vi "rsscope_core_global.vi"() -> ()   [LabVIEW 2014] (continued)
you see the signal that would be at the measurement point if the probe&apos;s input impedance is ideal (infinite impedance). Without removing the loading, you see the real signal at the measurement point, including the probe loading.\n\nAvailable Repeated Capabilities:\nChannel: CH1, CH2, CH3, CH4, CHExt\r\n\nRemote-control command(s):\nDEEMbedding<m>:COMPonent<n>:LOAD:REMProbeload"}, {"Level"=2, "Class Only"=FALSE, "Identifier"="RSSCOPE_ATTR_DEEMBEDDING_COMPONENT_IMPEDANCE_TYPE", "Descriptive Name"="Deembedding Component Impedance Type", "Data Type"=0, "Command"="DEEM{Channel}:COMP<Component>:LOAD", "Access"=2, "Range Table"="RsScope_rngDeembeddingComponentImpedanceType", "Read Callback"="rsscope_FormatDeembeddingComponentRepCapInt32_ReadCallback.vi", "Write Callback"="rsscope_FormatDeembeddingComponentRepCapInt32_WriteCallback.vi", "Supported Models"="", "Instrument Options"="K121", "Flags"=0, "Help"="Sets the impedance type of the DUT.\n\nAvailable Repeated Capabilities:\nChannel: CH1, CH2, CH3, CH4, CHExt\r\n\nRemote-control command(s):\nDEEMbedding<m>:COMPonent<n>:LOAD[:TYPE]"}, {"Level"=2, "Class Only"=FALSE, "Identifier"="RSSCOPE_ATTR_DEEMBEDDING_COMPONENT_IMPEDANCE", "Descriptive Name"="Deembedding Component Impedance", "Data Type"=1, "Command"="DEEM{Channel}:COMP<Component>:LOAD:IMP", "Access"=2, "Range Table"="", "Read Callback"="rsscope_FormatDeembeddingComponentRepCapReal64_ReadCallback.vi", "Write Callback"="rsscope_FormatDeembeddingComponentRepCapReal64_WriteCallback.vi", "Supported Models"="", "Instrument Options"="K121", "Flags"=0, "Help"="Impedance of the DUT. Shows the default source impedance or sets the user-defined constant impedance value. If an R&S RT-ZM probe is connected, the value depends on the selected probe mode: common mode, differential, or single-ended measurement.\n\nAvailable Repeated Capabilities:\nChannel: CH1, CH2, CH3, CH4, CHExt\r\n\nRemote-control command(s):\nDEEMbedding<m>:COMPonent<n>:LOAD:IMPedance"}, {"Level"=2, "Class Only"=FALSE, "Identifier"="RSSCOPE_ATTR_DEEMBEDDING_COMPONENT_IDENTICAL_PATHS", "Descriptive Name"="Deembedding Component Identical Paths", "Data Type"=3, "Command"="DEEM{Channel}:COMP<Component>:IDEN", "Access"=2, "Range Table"="", "Read Callback"="rsscope_FormatDeembeddingComponentRepCapBoolean_ReadCallback.vi", "Write Callback"="rsscope_FormatDeembeddingComponentRepCapBoolean_WriteCallback.vi", "Supported Models"="", "Instrument Options"="K121", "Flags"=0, "Help"="The setting is relevant if the measurement setup is a 4-port, and the component is a 2- port. Usually, these components are cables and adapters, which are described by *.s2p files. In case of a 4-port setup, 2 cables or 2 adapters are used. If they are identical, for example, when a matched-pair cable is used, they can be described by the same file. In this case, set the attribute to ON.\n\nAvailable Repeated Capabilities:\nChannel: CH1, CH2, CH3, CH4, CHExt\r\n\nRemote-control command(s):\nDEEMbedding<m>:COMPonent<n>:IDENtical"}, {"Level"=2, "Class Only"=FALSE, "Identifier"="RSSCOPE_ATTR_DEEMBEDDING_COMPONENT_INPUT_PORT_1", "Descriptive Name"="Deembedding Component Input Port 1", "Data Type"=0, "Command"="DEEM{Channel}:COMP<Component>:IPON", "Access"=2, "Range Table"="RsScope_rngDeembeddingComponentPort", "Read Callback"="rsscope_FormatDeembeddingComponentRepCapInt32_ReadCallback.vi", "Write Callback"="rsscope_FormatDeembeddingComponentRepCapInt32_WriteCallback.vi", "Supported Models"="", "Instrument Options"="K121", "Flags"=0, "Help"="Assign the ports to the input 1 of the component according to the data in the Touchstone file. This information is not directly written in the file. You need background information how the S-parameters were determined, i.e. which port was input and which port was output.\n\nAvailable Repeated Capabilities:\nChannel: CH1, CH2, CH3, CH4, CHExt\r\n\nRemote-control command(s):\nDEEMbedding<m>:COMPonent<n>:IPONe"}, {"Level"=2, "Class Only"=FALSE, "Identifier"="RSSCOPE_ATTR_DEEMBEDDING_COMPONENT_INPUT_PORT_2", "Descriptive Name"="Deembedding Component Input Port 2", "Data Type"=0, "Command"="DEEM{Channel}:COMP<Component>:IPTW", "Access"=2, "Range Table"="RsScope_rngDeembeddingComponentPort", "Read Callback"="rsscope_FormatDeembeddingComponentRepCapInt32_ReadCallback.vi", "Write Callback"="rsscope_FormatDeembeddingComponentRepCapInt32_WriteCallback.vi", "Supported Models"="", "Instrument Options"="K121", "Flags"=0, "Help"="Assign the ports to the input 2 of the component according to the data in the Touchstone file. This information is not directly written in the file. You need background information how the S-parameters were determined, i.e. which port was input and which port was output.\n\nAvailable Repeated Capabilities:\nChannel: CH1, CH2, CH3, CH4, CHExt\r\n\nRemote-control command(s):\nDEEMbedding<m>:COMPonent<n>:IPTWo"}, {"Level"=2, "Class Only"=FALSE, "Identifier"="RSSCOPE_ATTR_DEEMBEDDING_COMPONENT_OUTPUT_PORT_1", "Descriptive Name"="Deembedding Component Output Port 1", "Data Type"=0, "Command"="DEEM{Channel}:COMP<Component>:OPON", "Access"=2, "Range Table"="RsScope_rngDeembeddingComponentPort", "Read Callback"="rsscope_FormatDeembeddingComponentRepCapInt32_ReadCallback.vi", "Write Callback"="rsscope_FormatDeembeddingComponentRepCapInt32_WriteCallback.vi", "Supported Models"="", "Instrument Options"="K121", "Flags"=0, "Help"="Assign the ports to the output 1 of the component according to the data in the Touchstone file. This information is not directly written in the file. You need background information how the S-parameters were determined, i.e. which port was input and which port was output.\n\nAvailable Repeated Capabilities:\nChannel: CH1, CH2, CH3, CH4, CHExt\r\n\nRemote-control command(s):\nDEEMbedding<m>:COMPonent<n>:OPONe"}, {"Level"=2, "Class Only"=FALSE, "Identifier"="RSSCOPE_ATTR_DEEMBEDDING_COMPONENT_OUTPUT_PORT_2", "Descriptive Name"="Deembedding Component Output Port 2", "Data Type"=0, "Command"="DEEM{Channel}:COMP<Component>:OPTW", "Access"=2, "Range Table"="RsScope_rngDeembeddingComponentPort", "Read Callback"="rsscope_FormatDeembeddingComponentRepCapInt32_ReadCallback.vi", "Write Callback"="rsscope_FormatDeembeddingComponentRepCapInt32_WriteCallback.vi", "Supported Models"="", "Instrument Options"="K121", "Flags"=0, "Help"="Assign the ports to the output 2 of the component according to the data in the Touchstone file. This information is not directly written in the file. You need background information how the S-parameters were determined, i.e. which port was input and which port was output.\n\nAvailable Repeated Capabilities:\nChannel: CH1, CH2, CH3, CH4, CHExt\r\n\nRemote-control command(s):\nDEEMbedding<m>:COMPonent<n>:OPTWo"}, {"Level"=2, "Class Only"=FALSE, "Identifier"="RSSCOPE_ATTR_DEEMBEDDING_ATTENUATION_DC", "Descriptive Name"="Deembedding Attenuation DC", "Data Type"=1, "Command"="DEEM{Channel}:CADC?", "Access"=0, "Range Table"="", "Read Callback"="", "Write Callback"="", "Supported Models"="", "Instrument Options"="K121", "Flags"=0, "Help"="Maximum attenuation or gain of the measurement setup before deembedding at DC. This value is the expected basic attenuation or gain, which is corrected by deembedding.\n\nAvailable Repeated Capabilities:\nChannel: CH1, CH2, CH3, CH4, CHExt\r\n\nRemote-control command(s):\nDEEMbedding<m>:CADC?"}, {"Level"=2, "Class Only"=FALSE, "Identifier"="RSSCOPE_ATTR_DEEMBEDDING_ATTENUATION_MAX", "Descriptive Name"="Deembedding Attenuation Max", "Data Type"=1, "Command"="DEEM{Channel}:MATT?", "Access"=0, "Range Table"="", "Read Callback"="", "Write Callback"="", "Supported Models"="", "Instrument Options"="K121", "Flags"=0, "Help"="Maximum attenuation of the measurement setup before deembedding, with reference to a frequency response normalized at DC to 0 dB. The deembedding filter must amplify the amplitude response by the &apos;Attmax&apos; value, and thus also increases the noise by this value. The value also helps to decide whether deembedding is useful for the defined effective bandwidth.\n\nAvailable Repeated Capabilities:\nChannel: CH1, CH2, CH3, CH4, CHExt\r\n\nRemote-control command(s):\nDEEMbedding<m>:MATTenuation?"}, {"Level"=2, "Class Only"=FALSE, "Identifier"="RSSCOPE_ATTR_DEEMBEDDING_GAIN_MAX", "Descriptive Name"="Deembedding Gain Max", "Data Type"=1, "Command"="DEEM{Channel}:MGA?", "Access"=0, "Range Table"="", "Read Callback"="", "Write Callback"="", "Supported Models"="", "Instrument Options"="K121", "Flags"=0, "Help"="Maximum gain of the measurement setup before deembedding, with reference to a frequency response normalized at DC to 0dB. The deembedding filter must attenuate the amplitude response by this value. The value helps also to avoid an overload of the ADC.\n\nAvailable Repeated Capabilities:\nChannel: CH1, CH2, CH3, CH4, CHExt\r\n\nRemote-control command(s):\nDEEMbedding<m>:MGAin?"}, {"Level"=1, "Class Only"=TRUE, "Identifier"="", "Descriptive Name"="Mixed Signal Option (MSO)", "Data Type"=0, "Command"="", "Access"=0, "Range Table"="", "Read Callback"="", "Write Callback"="", "Supported Models"="", "Instrument Options"="", "Flags"=0, "Help"="The Mixed Signal Option R&S RTO-B1 adds logic analyzer functions to the classical\noscilloscope functions. Using the MSO option, you can analyze and debug embedded\nsystems with mixed-signal designs that use analog signals and correlated digital signals\nsimultaneously."}, {"Level"=2, "Class Only"=TRUE, "Identifier"="", "Descriptive Name"="Trigger", "Data Type"=0, "Command"="", "Access"=0, "Range Table"="", "Read Callback"="", "Write Callback"="", "Supported Models"="", "Instrument Options"="", "Flags"=0, "Help"="MSO trigger settings."}, {"Level"=3, "Class Only"=FALSE, "Identifier"="RSSCOPE_ATTR_MSO_TRIGGER_TYPE", "Descriptive Name"="MSO Trigger Type", "Data Type"=0, "Command"="TRIG:PAR:TYPE", "Access"=2, "Range Table"="rsscope_rngMSOTriggerType", "Read Callback"="", "Write Callback"="", "Supported Models"="", "Instrument Options"="B1", "Flags"=0, "Help"="Sets the MSO trigger type.\n\nAvailable Repeated Capabilities:\nNone\n\nRemote-control command(s):\nTRIGger<m>:PARallel:TYPE"}, {"Level"=3, "Class Only"=FALSE, "Identifier"="RSSCOPE_ATTR_MSO_TRIGGER_SOURCE", "Descriptive Name"="MSO Trigger Source", "Data Type"=0, "Command"="TRIG:SOUR", "Access"=2, "Range Table"="rsscope_rngMSOTriggerSource", "Read Callback"="", "Write Callback"="", "Supported Models"="", "Instrument Options"="B1", "Flags"=0, "Help"="Sets the trigger source for the selected trigger type.\n\nAvailable Repeated Capabilities:\nNone\n\nRemote-control command(s):\nTRIGger<m>:SOURce[:SELect]"}, {"Level"=3, "Class Only"=TRUE, "Identifier"="", "Descriptive Name"="Edge", "Data Type"=0, "Command"="", "Access"=0, "Range Table"="", "Read Callback"="", "Write Callback"="", "Supported Models"="", "Instrument Options"="", "Flags"=0, "Help"="MSO trigger edge settings."}, {"Level"=4, "Class Only"=FALSE, "Identifier"="RSSCOPE_ATTR_MSO_EDGE_TRIGGER_EXPRESSION", "Descriptive Name"="MSO Edge Trigger Expression", "Data Type"=2, "Command"="TRIGger1:PAR:EDGE:EXPR", "Access"=2, "Range Table"="", "Read Callback"="", "Write Callback"="", "Supported Models"="", "Instrument Options"="B1", "Flags"=0, "Help"="Defines a logical combination of several digital channels as trigger condition.\n\nExample: &apos;D1 and D2&apos;\n\nAvailable Repeated Capabilities:\nNone\n\nRemote-control command(s):\nTRIGger<m>:PARallel:EDGE:EXPRession[:DEFine]"}, {"Level"=4, "Class Only"=FALSE, "Identifier"="RSSCOPE_ATTR_MSO_EDGE_TRIGGER_SLOPE", "Descriptive Name"="MSO Edge Trigger Slope", "Data Type"=0, "Command"="TRIG:PAR:EDGE:SLOP", "Access"=2, "Range Table"="rsscope_rngTriggerSlope", "Read Callback"="", "Write Callback"="", "Supported Models"="", "Instrument Options"="B1", "Flags"=0, "Help"="Defines the edge - the state transition - of the signal to trigger on a single digital channel (a logic bit), or a logical combination of digital channels.\n\nAvailable Repeated Capabilities:\nNone\n\nRemote-control command(s):\nTRIGger<m>:PARallel:EDGE:SLOPe"}, {"Level"=3, "Class Only"=TRUE, "Identifier"="", "Descriptive Name"="Width", "Data Type"=0, "Command"="", "Access"=0, "Range Table"="", "Read Callback"="", "Write Callback"="", "Supported Models"="", "Instrument Options"="", "Flags"=0, "Help"="MSO trigger width settings."}, {"Level"=4, "Class Only"=FALSE, "Identifier"="RSSCOPE_ATTR_MSO_WIDTH_TRIGGER_EXPRESSION", "Descriptive Name"="MSO Width Trigger Expression", "Data Type"=2, "Command"="TRIGger1:PAR:WIDT:EXPR", "Access"=2, "Range Table"="", "Read Callback"="", "Write Callback"="", "Supported Models"="", "Instrument Options"="B1", "Flags"=0, "Help"="Defines a logical combination of several digital channels as trigger condition.\n\nExample: &apos;D1 and D2&apos;\n\nAvailable Repeated Capabilities:\nNone\n\nRemote-control command(s):\nTRIGger<m>:PARallel:WIDTh:EXPRession[:DEFine]"}, {"Level"=4, "Class Only"=FALSE, "Identifier"="RSSCOPE_ATTR_MSO_WIDTH_TRIGGER_POLARITY", "Descriptive Name"="MSO Width Trigger Polarity", "Data Type"=0, "Command"="TRIGger1:PAR:WIDT:POL", "Access"=2, "Range Table"="rsscope_rngTriggerSlope", "Read Callback"="", "Write Callback"="", "Supported Models"="", "Instrument Options"="B1", "Flags"=0, "Help"="Sets the polarity of the pulse. When triggering on a positive pulse, the trigger event occurs on the high to low transition of the pulse if the timing condition is true. When triggering on a negative pulse, the trigger event occurs on the low to high transition of the pulse if the timing condition is true.\n\nAvailable Repeated Capabilities:\nNone\n\nRemote-control command(s):\nTRIGger<m>:PARallel:WIDTh:POLarity"}, {"Level"=4, "Class Only"=FALSE, "Identifier"="RSSCOPE_ATTR_MSO_WIDTH_TRIGGER_CONDITION", "Descriptive Name"="MSO Width Trigger Condition", "Data Type"=0, "Command"="TRIGger1:PAR:WIDT:RANG", "Access"=2, "Range Table"="rsscope_rngWidthCondition", "Read Callback"="", "Write Callback"="", "Supported Models"="", "Instrument Options"="B1", "Flags"=0, "Help"="Selects how the range of a pulse width is defined.\n\nAvailable Repeated Capabilities:\nNone\n\nRemote-control command(s):\nTRIGger<m>:PARallel:WIDTh:RANGe"}, {"Level"=4, "Class Only"=FALSE, "Identifier"="RSSCOPE_ATTR_MSO_WIDTH_TRIGGER_WIDTH", "Descriptive Name"="MSO Width Trigger Width", "Data Type"=1, "Command"="TRIGger1:PAR:WIDT:WIDT", "Access"=2, "Range Table"="rsscope_rngMSOWidth", "Read Callback"="", "Write Callback"="", "Supported Models"="", "Instrument Options"="B1", "Flags"=0, "Help"="For the ranges &apos;Within&apos; and &apos;Outside&apos;, the width defines the center of a range which is defined by the limits &apos;+/-Delta&apos;. For the ranges &apos;Shorter&apos; and &apos;Longer&apos;, the width defines the maximum and minimum pulse width, respectively.\n\nAvailable Repeated Capabilities:\nNone\n\nRemote-control command(s):\nTRIGger<m>:PARallel:WIDTh:WIDTh"}, {"Level"=4, "Class Only"=FALSE, "Identifier"="RSSCOPE_ATTR_MSO_WIDTH_TRIGGER_DELTA", "Descriptive Name"="MSO Width Trigger Delta", "Data Type"=1, "Command"="TRIGger1:PAR:WIDT:DELT", "Access"=2, "Range Table"="rsscope_rngMSOWidthDelta", "Read Callback"="", "Write Callback"="", "Supported Models"="", "Instrument Options"="B1", "Flags"=0, "Help"="Defines a range around the width value.\n\nAvailable Repeated Capabilities:\nNone\n\nRemote-control command(s):\nTRIGger<m>:PARallel:WIDTh:DELTa"}, {"Level"=3, "Class Only"=TRUE, "Identifier"="", "Descriptive Name"="Timeout", "Data Type"=0, "Command"="", "Access"=0, "Range Table"="", "Read Callback"="", "Write Callback"="", "Supported Models"="", "Instrument Options"="", "Flags"=0, "Help"="MSO trigger timeout settings."}, {"Level"=4, "Class Only"=FALSE, "Identifier"="RSSCOPE_ATTR_MSO_TIMEOUT_TRIGGER_EXPRESSION", "Descriptive Name"="MSO Timeout Trigger Expression", "Data Type"=2, "Command"="TRIGger1:PAR:TIM:EXPR", "Access"=2, "Range Table"="", "Read Callback"="", "Write Callback"="", "Supported Models"="", "Instrument Options"="B1", "Flags"=0, "Help"="Defines a logical combination of several digital channels as trigger condition.\n\nExample: &apos;D1 and D2&apos;\n\nAvailable Repeated Capabilities:\nNone\n\nRemote-control command(s):\nTRIGger<m>:PARallel:TIMeout:EXPRession[:DEFine]"}, {"Level"=4, "Class Only"=FALSE, "Identifier"="RSSCOPE_ATTR_MSO_TIMEOUT_TRIGGER_VALUE", "Descriptive Name"="MSO Timeout Trigger Value", "Data Type"=1, "Command"="TRIGger1:PAR:TIM:TIME", "Access"=2, "Range Table"="rsscope_rngMSOTimeoutPattern", "Read Callback"="", "Write Callback"="", "Supported Models"="", "Instrument Options"="B1", "Flags"=0, "Help"="Defines the time limit for the timeout at which the instrument triggers.\n\nAvailable Repeated Capabilities:\nNone\n\nRemote-control command(s):\nTRIGger<m>:PARallel:TIMeout:TIME"}, {"Level"=4, "Class Only"=FALSE, "Identifier"="RSSCOPE_ATTR_MSO_TIMEOUT_TRIGGER_CONDITION", "Descriptive Name"="MSO Timeout Trigger Condition", "Data Type"=0, "Command"="TRIGger1:PAR:TIM:RANG", "Access"=2, "Range Table"="rsscope_rngMSOTimeoutCondition", "Read Callback"="", "Write Callback"="", "Supported Models"="", "Instrument Options"="B1", "Flags"=0, "Help"="Defines the relation of the signal level to the trigger level.\n\nAvailable Repeated Capabilities:\nNone\n\nRemote-control command(s):\nTRIGger<m>:PARallel:TIMeout:RANGe"}, {"Level"=3, "Class Only"=TRUE, "Identifier"="", "Descriptive Name"="Data2Clock", "Data Type"=0, "Command"="", "Access"=0, "Range Table"="", "Read Callback"="", "Write Callback"="", "Supported Models"="", "Instrument Options"="", "Flags"=0, "Help"="MSO trigger Data2Clock settings."}, {"Level"=4, "Class Only"=FALSE, "Identifier"="RSSCOPE_ATTR_MSO_DATA2CLOCK_TRIGGER_CLOCK_SOURCE", "Descriptive Name"="MSO Data2Clock Trigger Clock Source", "Data Type"=0, "Command"="TRIG1:PAR:SETH:CSO", "Access"=2, "Range Table"="rsscope_rngMSOClockSource", "Read Callback"="", "Write Callback"="", "Supported Models"="", "Instrument Options"="B1", "Flags"=0, "Help"="Sets the clock signal source.\n\nAvailable Repeated Capabilities:\nNone\n\nRemote-control command(s):\nTRIGger<m>:PARallel:SETHold:CSOurce[:VALue]"}, {"Level"=4, "Class Only"=FALSE, "Identifier"="RSSCOPE_ATTR_MSO_DATA2CLOCK_TRIGGER_CLOCK_EDGE", "Descriptive Name"="MSO Data2Clock Trigger Clock Edge", "Data Type"=0, "Command"="TRIG1:PAR:SETH:CSO:EDGE", "Access"=2, "Range Table"="rsscope_rngTriggerSlope", "Read Callback"="", "Write Callback"="", "Supported Models"="", "Instrument Options"="B1", "Flags"=0, "Help"="Sets the edge of the clock signal to define the time reference point for the setup and hold time.\n\nAvailable Repeated Capabilities:\nNone\n\nRemote-control command(s):\nTRIGger<m>:PARallel:SETHold:CSOurce:EDGE"}, {"Level"=4, "Class Only"=FALSE, "Identifier"="RSSCOPE_ATTR_MSO_DATA2CLOCK_TRIGGER_HOLD_TIME", "Descriptive Name"="MSO Data2Clock Trigger Hold Time", "Data Type"=1, "Command"="TRIG1:PAR:SETH:HTIM", "Access"=2, "Range Table"="rsscope_rngMSOData2ClockTime", "Read Callback"="", "Write Callback"="", "Supported Models"="", "Instrument Options"="B1", "Flags"=0, "Help"="Sets the minimum time after the clock edge while the data signal must stay steady above or below the data level. The hold time can be negative. In this case, the setup time is always positive. The setup/hold interval starts before the clock edge (setup time) and ends before the clock edge (hold time). If you change the negative hold time, the setup time is adjusted by the intrument.\n\nAvailable Repeated Capabilities:\nNone\n\nRemote-control command(s):\nTRIGger<m>:PARallel:SETHold:HTIMe"}, {"Level"=4, "Class Only"=FALSE, "Identifier"="RSSCOPE_ATTR_MSO_DATA2CLOCK_TRIGGER_SETUP_TIME", "Descriptive Name"="MSO Data2Clock Trigger SetupTime", "Data Type"=1, "Command"="TRIG1:PAR:SETH:STIM", "Access"=2, "Range Table"="rsscope_rngMSOData2ClockTime", "Read Callback"="", "Write Callback"="", "Supported Models"="", "Instrument Options"="B1", "Flags"=0, "Help"="Sets the minimum time before the clock edge while the data signal must stay steady above or below the data level. The setup time can be negative. In this case, the hold time is always positive. The setup/hold interval starts after the clock edge (setup time) and ends after the clock edge (hold time). If you change the negative setup time, the hold time is adjusted by the intrument.\n\nAvailable Repeated Capabilities:\nNone\n\nRemote-control command(s):\nTRIGger<m>:PARallel:SETHold:STIMe"}, {"Level"=3, "Class Only"=TRUE, "Identifier"="", "Descriptive Name"="State", "Data Type"=0, "Command"="", "Access"=0, "Range Table"="", "Read Callback"="", "Write Callback"="", "Supported Models"="", "Instrument Options"="", "Flags"=0, "Help"="MSO trigger state settings."}, {"Level"=4, "Class Only"=FALSE, "Identifier"="RSSCOPE_ATTR_MSO_STATE_TRIGGER_EXPRESSION", "Descriptive Name"="MSO State Trigger Expression", "Data Type"=2, "Command"="TRIGger1:PAR:STAT:EXPR", "Access"=2, "Range Table"="", "Read Callback"="", "Write Callback"="", "Supported Models"="", "Instrument Options"="B1", "Flags"=0, "Help"="Defines a logical combination of several digital channels as trigger condition.\n\nExample: &apos;D1 and D2&apos;\n\nAvailable Repeated Capabilities:\nNone\n\nRemote-control command(s):\nTRIGger<m>:PARallel:STATe:EXPRession[:DEFine]"}, {"Level"=4, "Class Only"=FALSE, "Identifier"="RSSCOPE_ATTR_MSO_STATE_TRIGGER_CLOCK_SOURCE", "Descriptive Name"="MSO State Trigger Clock Source", "Data Type"=0, "Command"="TRIGger1:PAR:STAT:CSO:VAL", "Access"=2, "Range Table"="rsscope_rngMSOClockSource", "Read Callback"="", "Write Callback"="", "Supported Models"="", "Instrument Options"="B1", "Flags"=0, "Help"="Sets the clock signal source.\n\nAvailable Repeated Capabilities:\nNone\n\nRemote-control command(s):\nTRIGger<m>:PARallel:STATe:CSOurce:VALue"}, {"Level"=4, "Class Only"=FALSE, "Identifier"="RSSCOPE_ATTR_MSO_STATE_TRIGGER_CLOCK_EDGE", "Descriptive Name"="MSO State Trigger Clock Edge", "Data Type"=0, "Command"="TRIGger1:PAR:STAT:CSO:EDGE", "Access"=2, "Range Table"="rsscope_rngTriggerSlope", "Read Callback"="", "Write Callback"="", "Supported Models"="", "Instrument Options"="B1", "Flags"=0, "Help"="Sets the edge of the clock signal. The crossing of the clock edge and the logical threshold defines the time at which the logical states and the bus value are analyzed.\n\nAvailable Repeated Capabilities:\nNone\n\nRemote-control command(s):\nTRIGger<m>:PARallel:STATe:CSOurce:EDGE"}, {"Level"=4, "Class Only"=TRUE, "Identifier"="", "Descriptive Name"="Digital Channel", "Data Type"=0, "Command"="", "Access"=0, "Range Table"="", "Read Callback"="", "Write Callback"="", "Supported Models"="", "Instrument Options"="", "Flags"=0, "Help"="MSO trigger state digital channel settings."}, {"Level"=5, "Class Only"=FALSE, "Identifier"="RSSCOPE_ATTR_MSO_STATE_TRIGGER_CHANNEL_STATUS_BIT", "Descriptive Name"="MSO State Trigger Channel Status Bit", "Data Type"=0, "Command"="TRIGger1:PAR:STAT:BIT{DigitalChannel}", "Access"=2, "Range Table"="rsscope_rngMSOTriggerChannelState", "Read Callback"="", "Write Callback"="", "Supported Models"="", "Instrument Options"="B1", "Flags"=0, "Help"="Sets the required state for each digital channel that is used in the bus.\n\nAvailable Repeated Capabilities:\nDigitalChannel: D0, D1, D2, D3, D4, D5, D6, D7, D8, D9, D10, D11, D12, D13, D14, D15\r\n\nRemote-control command(s):\nTRIGger<m>:PARallel:STATe:BIT<n>"}, {"Level"=3, "Class Only"=TRUE, "Identifier"="", "Descriptive Name"="Pattern", "Data Type"=0, "Command"="", "Access"=0, "Range Table"="", "Read Callback"="", "Write Callback"="", "Supported Models"="", "Instrument Options"="", "Flags"=0, "Help"="MSO trigger patern settings."}, {"Level"=4, "Class Only"=FALSE, "Identifier"="RSSCOPE_ATTR_MSO_PATTERN_TRIGGER_EXPRESSION", "Descriptive Name"="MSO Pattern Trigger Expression", "Data Type"=2, "Command"="TRIGger1:PAR:PATT:EXPR", "Access"=2, "Range Table"="", "Read Callback"="", "Write Callback"="", "Supported Models"="", "Instrument Options"="B1", "Flags"=0, "Help"="Defines a logical combination of several digital channels as trigger condition.\n\nExample: &apos;D1 and D2&apos;\n\nAvailable Repeated Capabilities:\nNone\n\nRemote-control command(s):\nTRIGger<m>:PARallel:PATTern:EXPRession[:DEFine]"}, {"Level"=4, "Class Only"=FALSE, "Identifier"="RSSCOPE_ATTR_MSO_PATTERN_TRIGGER_MODE", "Descriptive Name"="MSO Pattern Trigger Mode", "Data Type"=0, "Command"="TRIGger1:PAR:PATT:MODE", "Access"=2, "Range Table"="rsscope_rngMSOPatternMode", "Read Callback"="", "Write Callback"="", "Supported Models"="", "Instrument Options"="B1", "Flags"=0, "Help"="Sets the mode of the timing condition.\n\nAvailable Repeated Capabilities:\nNone\n\nRemote-control command(s):\nTRIGger<m>:PARallel:PATTern:MODE"}, {"Level"=4, "Class Only"=FALSE, "Identifier"="RSSCOPE_ATTR_MSO_PATTERN_TRIGGER_TIMEOUT_MODE", "Descriptive Name"="MSO Pattern Trigger Timeout Mode", "Data Type"=0, "Command"="TRIGger1:PAR:PATT:TIM:MODE", "Access"=2, "Range Table"="rsscope_rngMSOPatternTimeoutMode", "Read Callback"="", "Write Callback"="", "Supported Models"="", "Instrument Options"="B1", "Flags"=0, "Help"="Sets the state condition for the timeout qualification.\n\nAvailable Repeated Capabilities:\nNone\n\nRemote-control command(s):\nTRIGger<m>:PARallel:PATTern:TIMeout:MODE"}, {"Level"=4, "Class Only"=FALSE, "Identifier"="RSSCOPE_ATTR_MSO_PATTERN_TRIGGER_TIMEOUT", "Descriptive Name"="MSO Pattern Trigger Timeout", "Data Type"=1, "Command"="TRIGger1:PAR:PATT:TIM", "Access"=2, "Range Table"="rsscope_rngMSOTimeoutPattern", "Read Callback"="", "Write Callback"="", "Supported Models"="", "Instrument Options"="B1", "Flags"=0, "Help"="Defines how long the result of the pattern condition must be true or false.\n\nAvailable Repeated Capabilities:\nNone\n\nRemote-control command(s):\nTRIGger<m>:PARallel:PATTern:TIMeout[:TIME]"}, {"Level"=4, "Class Only"=FALSE, "Identifier"="RSSCOPE_ATTR_MSO_PATTERN_TRIGGER_WIDTH", "Descriptive Name"="MSO Pattern Trigger Width", "Data Type"=1, "Command"="TRIGger1:PAR:PATT:WIDT", "Access"=2, "Range Table"="rsscope_rngMSOTimeoutPattern", "Read Callback"="", "Write Callback"="", "Supported Models"="", "Instrument Options"="B1", "Flags"=0, "Help"="For the ranges &apos;Within&apos; and &apos;Outside&apos;, the width defines the center of a range which is defined by the limits &apos;Delta&apos;.\nFor the ranges &apos;Shorter&apos; and &apos;Longer&apos;, the width defines the maximum and minimum pulse width, respectively.\n\nAvailable Repeated Capabilities:\nNone\n\nRemote-control command(s):\nTRIGger<m>:PARallel:PATTern:WIDTh[:WIDTh]"}, {"Level"=4, "Class Only"=FALSE, "Identifier"="RSSCOPE_ATTR_MSO_PATTERN_TRIGGER_DELTA", "Descriptive Name"="MSO Pattern Trigger Delta", "Data Type"=1, "Command"="TRIGger1:PAR:PATT:WIDT:DELT", "Access"=2, "Range Table"="rsscope_rngMSOWidthDelta", "Read Callback"="", "Write Callback"="", "Supported Models"="", "Instrument Options"="B1", "Flags"=0, "Help"="Defines how the range of a pulse width is defined for keeping up the true result of the pattern condition.\n\nAvailable Repeated Capabilities:\nNone\n\nRemote-control command(s):\nTRIGger<m>:PARallel:PATTern:WIDTh:DELTa"}, {"Level"=4, "Class Only"=FALSE, "Identifier"="RSSCOPE_ATTR_MSO_PATTERN_TRIGGER_CONDITION", "Descriptive Name"="MSO Pattern Trigger Condition", "Data Type"=0, "Command"="TRIGger1:PAR:PATT:WIDT:RANG", "Access"=2, "Range Table"="rsscope_rngWidthCondition", "Read Callback"="", "Write Callback"="", "Supported Models"="", "Instrument Options"="B1", "Flags"=0, "Help"="Defines how the range of a pulse width is defined for keeping up the true result of the pattern condition.\n\nAvailable Repeated Capabilities:\nNone\n\nRemote-control command(s):\nTRIGger<m>:PARallel:PATTern:WIDTh:RANGe"}, {"Level"=4, "Class Only"=TRUE, "Identifier"="", "Descriptive Name"="Digital Channel", "Data Type"=0, "Command"="", "Access"=0, "Range Table"="", "Read Callback"="", "Write Callback"="", "Supported Models"="", "Instrument Options"="", "Flags"=0, "Help"="MSO trigger patern digital channel settings."}, {"Level"=5, "Class Only"=FALSE, "Identifier"="RSSCOPE_ATTR_MSO_PATTERN_TRIGGER_CHANNEL_STATUS_BIT", "Descriptive Name"="MSO Pattern Trigger Channel Status Bit", "Data Type"=0, "Command"="TRIGger1:PAR:PATT:BIT{DigitalChannel}", "Access"=2, "Range Table"="rsscope_rngMSOTriggerChannelState", "Read Callback"="", "Write Callback"="", "Supported Models"="", "Instrument Options"="B1", "Flags"=0, "Help"="Sets the required state for each digital channel that is used in the bus.\n\nAvailable Repeated Capabilities:\nDigitalChannel: D0, D1, D2, D3, D4, D5, D6, D7, D8, D9, D10, D11, D12, D13, D14, D15\r\n\nRemote-control command(s):\nTRIGger<m>:PARallel:PATTern:BIT<n>"}, {"Level"=3, "Class Only"=TRUE, "Identifier"="", "Descriptive Name"="Serial Pattern", "Data Type"=0, "Command"="", "Access"=0, "Range Table"="", "Read Callback"="", "Write Callback"="", "Supported Models"="", "Instrument Options"="", "Flags"=0, "Help"="MSO trigger serial pattern settings."}, {"Level"=4, "Class Only"=FALSE, "Identifier"="RSSCOPE_ATTR_MSO_SERIAL_PATTERN_TRIGGER_EXPRESSION", "Descriptive Name"="MSO Serial Pattern Trigger Expression", "Data Type"=2, "Command"="TRIGger1:PAR:SPAT:EXPR", "Access"=2, "Range Table"="", "Read Callback"="", "Write Callback"="", "Supported Models"="", "Instrument Options"="B1", "Flags"=0, "Help"="Defines a logical combination of several digital channels as trigger condition.\n\nExample: &apos;D1 and D2&apos;\n\nAvailable Repeated Capabilities:\nNone\n\nRemote-control command(s):\nTRIGger<m>:PARallel:SPATtern:EXPRession[:DEFine]"}, {"Level"=4, "Class Only"=FALSE, "Identifier"="RSSCOPE_ATTR_MSO_SERIAL_PATTERN_TRIGGER_CLOCK_SOURCE", "Descriptive Name"="MSO Serial Pattern Trigger Clock Source", "Data Type"=0, "Command"="TRIGger1:PAR:SPAT:CSO:VAL", "Access"=2, "Range Table"="rsscope_rngMSOClockSource", "Read Callback"="", "Write Callback"="", "Supported Models"="", "Instrument Options"="B1", "Flags"=0, "Help"="Sets the clock signal source.\n\nAvailable Repeated Capabilities:\nNone\n\nRemote-control command(s):\nTRIGger<m>:PARallel:SPATtern:CSOurce[:VALue]"}, {"Level"=4, "Class Only"=FALSE, "Identifier"="RSSCOPE_ATTR_MSO_SERIAL_PATTERN_TRIGGER_CLOCK_EDGE", "Descriptive Name"="MSO Serial Pattern Trigger Clock Edge", "Data Type"=0, "Command"="TRIGger1:PAR:SPAT:CSO:EDGE", "Access"=2, "Range Table"="rsscope_rngTriggerSlope", "Read Callback"="", "Write Callback"="", "Supported Models"="", "Instrument Options"="B1", "Flags"=0, "Help"="The clock edge defines the point in time when the state of the data signal is checked.\n\nAvailable Repeated Capabilities:\nNone\n\nRemote-control command(s):\nTRIGger<m>:PARallel:SPATtern:CSOurce:EDGE"}, {"Level"=4, "Class Only"=FALSE, "Identifier"="RSSCOPE_ATTR_MSO_SERIAL_PATTERN_TRIGGER_PATTERN", "Descriptive Name"="MSO Serial Pattern Trigger Pattern", "Data Type"=2, "Command"="TRIGger1:PAR:SPAT:PATT", "Access"=2, "Range Table"="", "Read Callback"="", "Write Callback"="", "Supported Models"="", "Instrument Options"="", "Flags"=0, "Help"="The pattern contains the bits of the serial data to be found in the data stream. The maximum length of the pattern is 128 bit. You can enter the pattern in binary or hexadecimal format.\n\nAvailable Repeated Capabilities:\nNone\n\nRemote-control command(s):\nTRIGger<m>:PARallel:SPATtern:PATTern"}, {"Level"=2, "Class Only"=TRUE, "Identifier"="", "Descriptive Name"="Digital Channel", "Data Type"=0, "Command"="", "Access"=0, "Range Table"="", "Read Callback"="", "Write Callback"="", "Supported Models"="", "Instrument Options"="", "Flags"=0, "Help"="Selects Digital Channel."}, {"Level"=3, "Class Only"=FALSE, "Identifier"="RSSCOPE_ATTR_MSO_SIGNAL_LABEL", "Descriptive Name"="MSO Signal Label", "Data Type"=2, "Command"="DIG{DigitalChannel}:LAB", "Access"=2, "Range Table"="", "Read Callback"="", "Write Callback"="", "Supported Models"="", "Instrument Options"="B1", "Flags"=0, "Help"="Selects and configure the digital channels that are used in the selected bus.\n\nAvailable Repeated Capabilities:\nDigitalChannel: D0, D1, D2, D3, D4, D5, D6, D7, D8, D9, D10, D11, D12, D13, D14, D15\r\n\nRemote-control command(s):\nDIGital<m>:LABel"}, {"Level"=3, "Class Only"=FALSE, "Identifier"="RSSCOPE_ATTR_MSO_DIGITAL_CHANNEL_DISPLAY", "Descriptive Name"="MSO Digital Channel Display", "Data Type"=3, "Command"="DIG{DigitalChannel}:DISP", "Access"=2, "Range Table"="", "Read Callback"="", "Write Callback"="", "Supported Models"="", "Instrument Options"="", "Flags"=0, "Help"="Enables or disables the indicated digital channel, displays it, and enables the parallel Bus1 if the bus was disabled. That is, RSSCOPE_ATTR_MSO_DISPLAY_SHOW_DIGITAL_SIGNALS and RSSCOPE_ATTR_MSO_BUS_STATE are set to ON automatically.\n\nIf another active bus already uses the selected digital channel, the instrument disables the other bus to avoid conflicts.\nFor Bus1, the DIG:DISP command has the same effect as RSSCOPE_ATTR_MSO_SIGNAL_ASSIGN_STATE. To enable digital channels for buses 2, 3 and 4, use the RSSCOPE_ATTR_MSO_SIGNAL_ASSIGN_STATE command.\n\nAvailable Repeated Capabilities:\nDigitalChannel: D0, D1, D2, D3, D4, D5, D6, D7, D8, D9, D10, D11, D12, D13, D14, D15\r\n\nRemote-control command(s):\nDIGital<m>:DISPlay"}, {"Level"=3, "Class Only"=FALSE, "Identifier"="RSSCOPE_ATTR_MSO_SIGNAL_DESKEW", "Descriptive Name"="MSO Signal Deskew", "Data Type"=1, "Command"="DIG{DigitalChannel}:DESK", "Access"=2, "Range Table"="rsscope_rngMSOSignalDeskew", "Read Callback"="", "Write Callback"="", "Supported Models"="", "Instrument Options"="B1", "Flags"=0, "Help"="Sets an individual delay for each digital channel to time-align it with other digital channels. The deskew value compensates delays that are known from the circuit specifics or caused by the different length of cables.\n\nAvailable Repeated Capabilities:\nDigitalChannel: D0, D1, D2, D3, D4, D5, D6, D7, D8, D9, D10, D11, D12, D13, D14, D15\r\n\nRemote-control command(s):\nDIGital<m>:DESKew"}, {"Level"=3, "Class Only"=FALSE, "Identifier"="RSSCOPE_ATTR_MSO_TECHNOLOGY", "Descriptive Name"="MSO Technology", "Data Type"=0, "Command"="DIG{DigitalChannel}:TECH", "Access"=2, "Range Table"="rsscope_rngProtocolTechnology", "Read Callback"="", "Write Callback"="", "Supported Models"="", "Instrument Options"="B1", "Flags"=0, "Help"="Selects the threshold voltage for various types of integrated circuits and applies it to all digital channels.\n\nAvailable Repeated Capabilities:\nDigitalChannel: D0, D1, D2, D3, D4, D5, D6, D7, D8, D9, D10, D11, D12, D13, D14, D15\r\n\nRemote-control command(s):\nDIGital<m>:TECHnology"}, {"Level"=3, "Class Only"=FALSE, "Identifier"="RSSCOPE_ATTR_MSO_TRESHOLD", "Descriptive Name"="MSO Treshold", "Data Type"=1, "Command"="DIG{DigitalChannel}:THR", "Access"=2, "Range Table"="", "Read Callback"="", "Write Callback"="", "Supported Models"="", "Instrument Options"="B1", "Flags"=0, "Help"="Sets the logical threshold for the indicated digital channel.\n\nAvailable Repeated Capabilities:\nDigitalChannel: D0, D1, D2, D3, D4, D5, D6, D7, D8, D9, D10, D11, D12, D13, D14, D15\r\n\nRemote-control command(s):\nDIGital<m>:THReshold"}, {"Level"=3, "Class Only"=FALSE, "Identifier"="RSSCOPE_ATTR_MSO_HYSTERESIS", "Descriptive Name"="MSO Hysteresis", "Data Type"=0, "Command"="DIG{DigitalChannel}:HYST", "Access"=2, "Range Table"="rsscope_rngMSOHysteresis", "Read Callback"="", "Write Callback"="", "Supported Models"="", "Instrument Options"="B1", "Flags"=0, "Help"="This control defines the size of the hysteresis to avoid the change of signal states due to noise.\n\nAvailable Repeated Capabilities:\nDigitalChannel: D0, D1, D2, D3, D4, D5, D6, D7, D8, D9, D10, D11, D12, D13, D14, D15\r\n\nRemote-control command(s):\nDIGital<m>:HYSTeresis"}, {"Level"=3, "Class Only"=FALSE, "Identifier"="RSSCOPE_ATTR_MSO_DIGITAL_CHANNEL_COUPLING", "Descriptive Name"="MSO Digital Channel Coupling", "Data Type"=3, "Command"="DIG:THC", "Access"=2, "Range Table"="", "Read Callback"="", "Write Callback"="", "Supported Models"="", "Instrument Options"="B1", "Flags"=0, "Help"="Sets the threshold and the hysteresis for all digital channels of parallel bus 1 to the same value. RSSCOPE_ATTR_MSO_CHANNEL_COUPLING is used to set all buses.\n\nAvailable Repeated Capabilities:\nNone\n\nRemote-control command(s):\nDIGital<m>:THCoupling"}, {"Level"=2, "Class Only"=TRUE, "Identifier"="", "Descriptive Name"="Parallel Bus", "Data Type"=0, "Command"="", "Access"=0, "Range Table"="", "Read Callback"="", "Write Callback"="", "Supported Models"="", "Instrument Options"="", "Flags"=0, "Help"="Selects Parallel Bus."}, {"Level"=3, "Class Only"=FALSE, "Identifier"="RSSCOPE_ATTR_MSO_BUS_STATE", "Descriptive Name"="MSO Bus State", "Data Type"=3, "Command"="BUS{SerialBus}:PAR:STAT", "Access"=2, "Range Table"="", "Read Callback"="", "Write Callback"="", "Supported Models"="", "Instrument Options"="B1", "Flags"=0, "Help"="Enables/disables the indicated parallel bus.\n\nAvailable Repeated Capabilities:\nSerialBus: SB1, SB2, SB3, SB4\r\n\nRemote-control command(s):\nBUS<m>:PARallel:STATe"}, {"Level"=3, "Class Only"=FALSE, "Identifier"="RSSCOPE_ATTR_MSO_DISPLAY_SHOW_DIGITAL_SIGNALS", "Descriptive Name"="MSO Display Show Digital Signals", "Data Type"=3, "Command"="BUS{SerialBus}:PAR:DISP:SHDI", "Access"=2, "Range Table"="", "Read Callback"="", "Write Callback"="", "Supported Models"="", "Instrument Options"="", "Flags"=0, "Help"="If enabled, the selected digital signals are shown in the diagram. Each channel is displayed as a logic signal.\n\nAvailable Repeated Capabilities:\nSerialBus: SB1, SB2, SB3, SB4\r\n\nRemote-control command(s):\nBUS<m>:PARallel:DISPlay:SHDI"}, {"Level"=3, "Class Only"=FALSE, "Identifier"="RSSCOPE_ATTR_MSO_DISPLAY_SHOW_BUS", "Descriptive Name"="MSO Display Show Bus", "Data Type"=3, "Command"="BUS{SerialBus}:PAR:DISP:SHBU", "Access"=2, "Range Table"="", "Read Callback"="", "Write Callback"="", "Supported Models"="", "Instrument Options"="", "Flags"=0, "Help"="Shows or hides the indicated parallel bus. If enabled, the resulting bus signal and bus values are displayed in the diagram.\n\nAvailable Repeated Capabilities:\nSerialBus: SB1, SB2, SB3, SB4\r\n\nRemote-control command(s):\nBUS<m>:PARallel:DISPlay:SHBU"}, {"Level"=3, "Class Only"=FALSE, "Identifier"="RSSCOPE_ATTR_MSO_DISPLAY_REPRESENTATION", "Descriptive Name"="MSO Display Representation", "Data Type"=0, "Command"="BUS{SerialBus}:PAR:DISP:BTYP", "Access"=2, "Range Table"="rsscope_rngMSODisplayRepresentation", "Read Callback"="", "Write Callback"="", "Supported Models"="", "Instrument Options"="B1", "Flags"=0, "Help"="Selects the display type of the indicated parallel bus.\n\nAvailable Repeated Capabilities:\nSerialBus: SB1, SB2, SB3, SB4\r\n\nRemote-control command(s):\nBUS<m>:PARallel:DISPlay:BTYP"}, {"Level"=3, "Class Only"=FALSE, "Identifier"="RSSCOPE_ATTR_MSO_CLOCKED_BUS_STATE", "Descriptive Name"="MSO Clocked Bus State", "Data Type"=3, "Command"="BUS{SerialBus}:PAR:CLON", "Access"=2, "Range Table"="", "Read Callback"="", "Write Callback"="", "Supported Models"="", "Instrument Options"="B1", "Flags"=0, "Help"="Defines if the bus is a clocked bus - one of the digital channels serves as clock of the bus.\n\nAvailable Repeated Capabilities:\nSerialBus: SB1, SB2, SB3, SB4\r\n\nRemote-control command(s):\nBUS<m>:PARallel:CLON"}, {"Level"=3, "Class Only"=FALSE, "Identifier"="RSSCOPE_ATTR_MSO_CLOCKED_BUS", "Descriptive Name"="MSO Clocked Bus", "Data Type"=0, "Command"="BUS{SerialBus}:PAR:CLOC", "Access"=2, "Range Table"="rsscope_rngMSOClockSource", "Read Callback"="", "Write Callback"="", "Supported Models"="", "Instrument Options"="B1", "Flags"=0, "Help"="Selects the digital channel used as clock of the indicated parallel bus.\n\nAvailable Repeated Capabilities:\nSerialBus: SB1, SB2, SB3, SB4\r\n\nRemote-control command(s):\nBUS<m>:PARallel:CLOCk"}, {"Level"=3, "Class Only"=FALSE, "Identifier"="RSSCOPE_ATTR_MSO_CLOCKED_BUS_SLOPE", "Descriptive Name"="MSO 
